vi "Convert Channel Settings to Analog.vi"(11 "channel settings":T1[](array[typedef])) -> (2 "channel default values":dbl[](array[numeric]), 3 "channel names":string[](array[string]))   [LabVIEW 2020, in "Scan Engine Scripting.lvlib"]
uses:
  Scan Engine Scripting.lvlib
  Modules/Mode Classes/Controls/analog channel settings.ctl
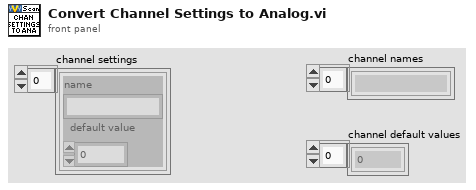
[diagram p1: front panel]
types:
  T1 = typedef "Scan Engine Scripting.lvlib/analog channel settings.ctl" = cluster{"name":string, "default value":dbl}
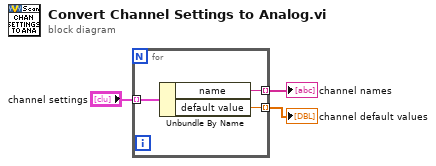
[diagram p0: block diagram]
diagram:
  n1 = for {
    tunnel: "channel settings" -> [w6] mode=indexing
    tunnel: [w5] -> w2 mode=indexing
    tunnel: [w4] -> w3 mode=indexing
    n2 = Unbundle By Name(w6) -> ("name"=w5:string, "default value"=w4:dbl)
  }
  "channel default values" <- w3
  "channel names" <- w2
